vi "GlobSave2File7.vi"(1 "Function select":string) -> (0 "stop":bool)   [LabVIEW 2013]
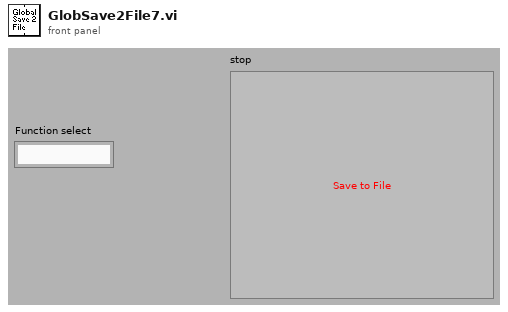
[diagram p1: front panel]
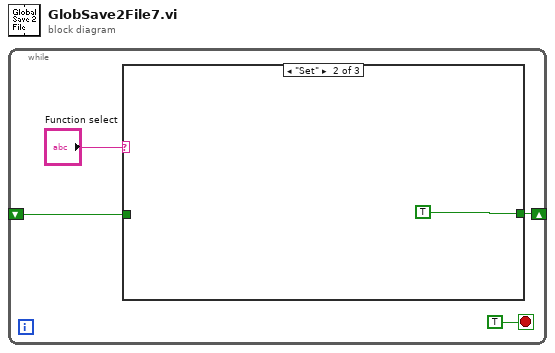
[diagram p0: block diagram]
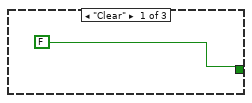
[diagram p2: hidden frame]
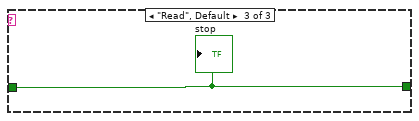
[diagram p3: hidden frame]
diagram:
  n1 = while {
    shift-right: [w2] -> _
    shift-left: _ -> [w1]
    stop <- TRUE stop-if-true
    n2 = case shown="\"Set\"" "Function select" {
      tunnel: [FALSE TRUE w7] -> w2
      tunnel: w1 -> [_ _ w7]
      frame "Clear" {
      }
      frame "Set" {
      }
      frame "Read", Default {
        "stop" <- w7
      }
    }
  }
